vi "Link Control References.vi"(8 "error in (no error)":errorcluster, 10 "Control Refs":T1[](array[typedef]), 11 "Instruments in":refnum<class "Instruments.lvclass">) -> (0 "error out":errorcluster, 3 "Instruments out":refnum<class "Instruments.lvclass">)   [LabVIEW 2023, in "Instruments.lvlib" / "Instruments.lvclass"]
doc: "This dynamically dispatched routine is meant to route any provided control references to class private references by name (label text)"
uses:
  Library/Instruments.lvclass
  C:/Users/Public/Documents/Development/builds/Framework/Actor Framework.lvlibp/1abvi3w/vi.lib/ActorFramework/Actor/Actor.lvclass
  builds/Framework/Engine.lvlibp/Engine/Custom Controls/Control Reference.ctl
  Library/Instruments.lvclass/Instruments.ctl
  0061f6fb-0229-4b67-9885-5618f8887638.vi
  builds/Framework/Actor Framework.lvlibp/1abvi3w/vi.lib/ActorFramework/Actor/Read Actor Label.vi
  <vilib>/Comparison/Equal/Equal Functor/Equal Functor.lvclass
  builds/Framework/Engine.lvlibp/Engine/Library/Engine.lvclass
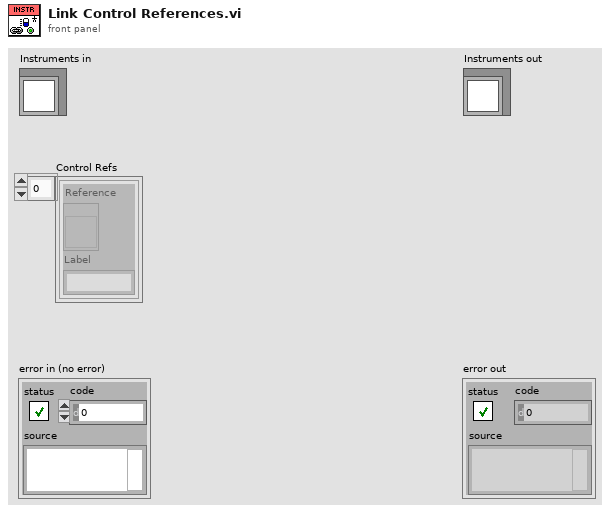
[diagram p1: front panel]
types:
  T1 = typedef "Engine.lvlibp/Engine.lvclass/Control Reference.ctl" = cluster{"Reference":refnum<vi>, "Label":string}
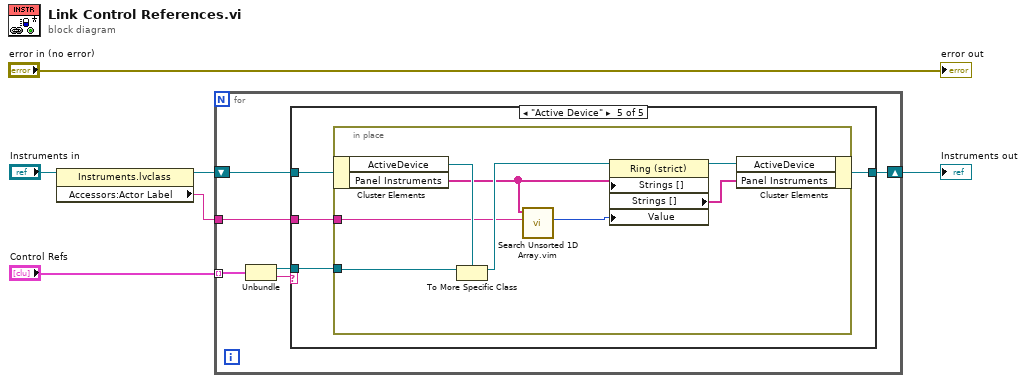
[diagram p0: block diagram]
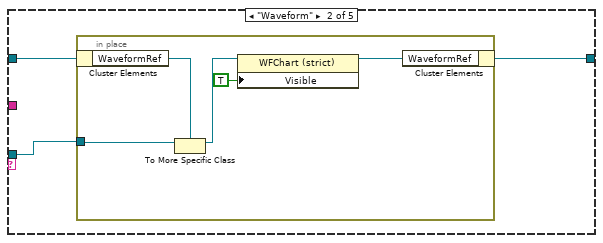
[diagram p3: hidden frame]
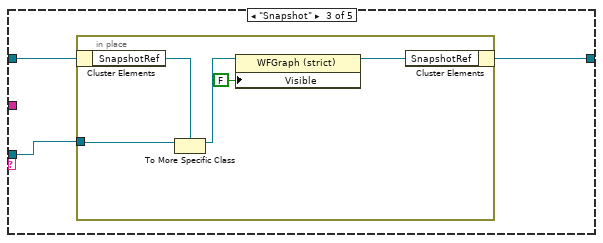
[diagram p4: hidden frame]
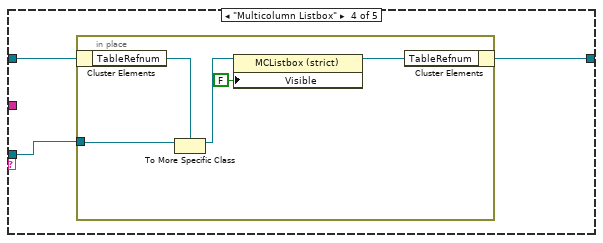
[diagram p5: hidden frame]
diagram:
  n1 = property class="Instruments.lvclass"(reference="Instruments in") -> (reference out=w2:refnum<class "Instruments.lvclass">, "Accessors:Actor Label"=w1:string)  [unwired: 1 in, 1 out]
  n2 = for {
    tunnel: "Control Refs" -> [w12] mode=indexing
    shift-right: [w8] -> w4
    shift-left: w2 -> [w9]
    tunnel: w1 -> [w7]
    n3 = Unbundle(w12) -> ("Reference"=w10:refnum<vi>, "Label"=w11:string)
    n4 = case shown="\"Active Device\"" w11 {
      tunnel: w10 -> [_ w14 w22 w30 w39]
      tunnel: w9 -> [w13 w16 w24 w32 w41]
      tunnel: [w13 w15 w23 w31 w40] -> w8
      tunnel: w7 -> [_ _ _ _ w38]
      frame "False", Default {
      }
      frame "Waveform" {
        n5 = in-place {
          in-place-border: w14 -> [w21]
          n6 = in-place-cluster #1(w16) -> ("WaveformRef"=w20:refnum<vi>)
          n7 = To More Specific Class(target class=w20, reference=w21) -> (specific class reference=w19:refnum<vi>)  [unwired: 1 in, 1 out]
          n8 = property class="WFChart (strict)"(reference=w19, "Visible"=TRUE) -> (reference out=w18:refnum<vi>)  [unwired: 1 in, 1 out]
          n9 = in-place-cluster #1("WaveformRef"=w18) -> (w15:refnum<class "Instruments.lvclass">)
        }
      }
      frame "Snapshot" {
        n10 = in-place {
          in-place-border: w22 -> [w29]
          n11 = in-place-cluster #2(w24) -> ("SnapshotRef"=w28:refnum<vi>)
          n12 = To More Specific Class(target class=w28, reference=w29) -> (specific class reference=w27:refnum<vi>)  [unwired: 1 in, 1 out]
          n13 = property class="WFGraph (strict)"(reference=w27, "Visible"=FALSE) -> (reference out=w26:refnum<vi>)  [unwired: 1 in, 1 out]
          n14 = in-place-cluster #2("SnapshotRef"=w26) -> (w23:refnum<class "Instruments.lvclass">)
        }
      }
      frame "Multicolumn Listbox" {
        n15 = in-place {
          in-place-border: w30 -> [w37]
          n16 = in-place-cluster #3(w32) -> ("TableRefnum"=w36:refnum<vi>)
          n17 = To More Specific Class(target class=w36, reference=w37) -> (specific class reference=w35:refnum<vi>)  [unwired: 1 in, 1 out]
          n18 = property class="MCListbox (strict)"(reference=w35, "Visible"=FALSE) -> (reference out=w34:refnum<vi>)  [unwired: 1 in, 1 out]
          n19 = in-place-cluster #3("TableRefnum"=w34) -> (w31:refnum<class "Instruments.lvclass">)
        }
      }
      frame "Active Device" {
        n20 = in-place {
          in-place-border: w39 -> [w49]
          in-place-border: w38 -> [w43]
          n21 = in-place-cluster #4(w41) -> ("ActiveDevice"=w48:refnum<vi>, "Panel Instruments"=w44:string[])
          n22 = To More Specific Class(target class=w48, reference=w49) -> (specific class reference=w47:refnum<vi>)  [unwired: 1 in, 1 out]
          n23 = call "Search Unsorted 1D Array.vim"("element"=w43, "unsorted 1D array"=w44) -> ("index of element"=w42:i32)  [unwired: 9 in]
          n24 = property class="Ring (strict)"(reference=w47, "Strings []"=w44, "Value"=w42) -> (reference out=w46:refnum<vi>, "Strings []"=w45:string[])  [unwired: 1 in, 1 out]
          n25 = in-place-cluster #4("ActiveDevice"=w46, "Panel Instruments"=w45) -> (w40:refnum<class "Instruments.lvclass">)
        }
      }
    }
  }
  "Instruments out" <- w4
  "error out" <- "error in (no error)"
